vi "Disabled.vi"(7 "Robot Mode":T2, 10 "Match Info":T1={"Autonomous Elapsed Seconds"=0.0, "TeleOp Elapsed Seconds"=0.0, "Disabled Elapsed Seconds"=0.0, "Visited Autonomous"=FALSE, "Visited TeleOp"=FALSE, "Visited Disabled"=FALSE, "Autonomous Settings"={"Autonomous Style"=enum."Independent", "VI Refnum"=refnum}}, 11 "Call Context":T3) -> ()   [LabVIEW 2012]
doc: "This VI is called each time a disabled packet is received from the DS. It is often used to prepare for the next robot mode, to calibrate sensors, etc."
uses:
  <vilib>/Rock Robotics/WPI/DriverStation/WPI_DriverStationDerivedRobotMode.ctl
  <vilib>/Rock Robotics/WPI/DriverStation/WPI_DriverStationRobotMode2.ctl
  <vilib>/Rock Robotics/WPI/DriverStation/WPI_DriverStationMatch Info.ctl
  Robot Global Data.vi
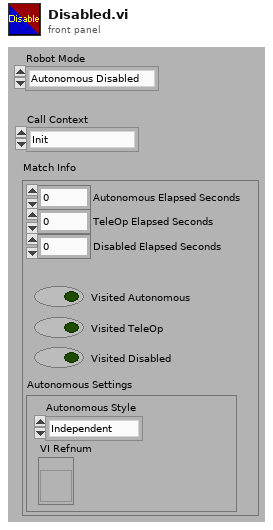
[diagram p1: front panel]
types:
  T1 = typedef "WPI_DriverStationMatch Info.ctl" = cluster{"Autonomous Elapsed Seconds":dbl, "TeleOp Elapsed Seconds":dbl, "Disabled Elapsed Seconds":dbl, "Visited Autonomous":bool, "Visited TeleOp":bool, "Visited Disabled":bool, "Autonomous Settings":cluster{"Autonomous Style":enum16{"Iterative", "Independent"}, "VI Refnum":refnum<vi>}}
  T2 = typedef "WPI_DriverStationRobotMode2.ctl" = enum16{"Autonomous Disabled", "Autonomous Enabled", "Teleop Disabled", "Teleop Enabled", "Timeout", "Finish", "Test Disabled", "Test Enabled"}
  T3 = typedef "WPI_DriverStationDerivedRobotMode.ctl" = enum16{"Init", "Execute", "Stop"}
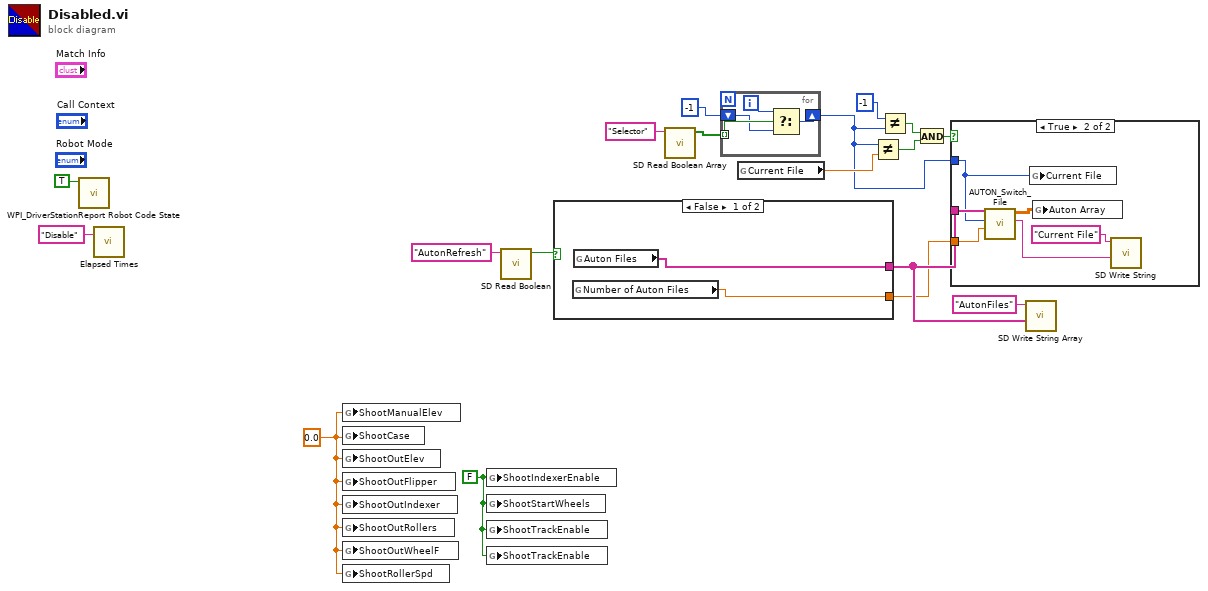
[diagram p0: block diagram]
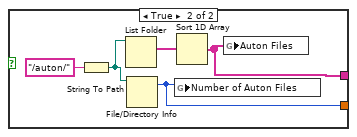
[diagram p3: hidden frame]
diagram:
  w13 = FALSE ("ShootIndexerEnable")
  w12 = 0.0 ("ShootCase")
  n1 = call <vilib>:"WPI_DriverStationReport Robot Code State.vi"("Disabled"=TRUE ("Autonomous")) -> ()  [unwired: 10 in, 1 out]
  n2 = call "Elapsed Times.vi"("Call Name"="Disable") -> ()  [unwired: 2 in, 1 out]
  n3 = global write "Robot Global Data.vi" "ShootManualElev"(w12) -> ()
  n4 = global write "Robot Global Data.vi" "ShootCase"(w12) -> ()
  n5 = global write "Robot Global Data.vi" "ShootOutElev"(w12) -> ()
  n6 = global write "Robot Global Data.vi" "ShootOutFlipper"(w12) -> ()
  n7 = global write "Robot Global Data.vi" "ShootOutIndexer"(w12) -> ()
  n8 = global write "Robot Global Data.vi" "ShootOutRollers"(w12) -> ()
  n9 = global write "Robot Global Data.vi" "ShootOutWheelF"(w12) -> ()
  n10 = global write "Robot Global Data.vi" "ShootRollerSpd"(w12) -> ()
  n11 = global write "Robot Global Data.vi" "ShootIndexerEnable"(w13) -> ()
  n12 = global write "Robot Global Data.vi" "ShootStartWheels"(w13) -> ()
  n13 = global write "Robot Global Data.vi" "ShootTrackEnable"(w13) -> ()
  n14 = global write "Robot Global Data.vi" "ShootTrackEnable"(w13) -> ()
  n15 = call <vilib>:"SD Read Boolean.vi"("Name"="AutonRefresh") -> ("Boolean"=w2:bool)  [unwired: 8 in, 2 out]
  n16 = case shown="False" w2 {
    tunnel: [w19 w22] -> w15
    tunnel: [w20 w21] -> w17
    frame False {
      n17 = global read "Robot Global Data.vi" "Number of Auton Files"() -> (w19:dbl)
      n18 = global read "Robot Global Data.vi" "Auton Files"() -> (w20:string[])
    }
    frame True {
      n19 = String To Path(string="/auton/") -> (path=w24:path)
      n20 = List Folder(path=w24) -> (filenames=w23:string[])  [unwired: 3 in, 3 out]
      n21 = File/Directory Info(path=w24) -> (size=w22:i64)  [unwired: 1 in, 6 out]
      n22 = global write "Robot Global Data.vi" "Number of Auton Files"(w22) -> ()
      n23 = Sort 1D Array(array=w23) -> (sorted array=w21:string[])
      n24 = global write "Robot Global Data.vi" "Auton Files"(w21) -> ()
    }
  }
  n25 = call <vilib>:"SD Read Boolean Array.vi"("Name"="Selector") -> ("Boolean Array"=w10:bool[])  [unwired: 8 in, 2 out]
  n26 = for {
    tunnel: w10 -> [w29] mode=indexing
    shift-right: [w27] -> w3
    shift-left: -1 -> [w26]
    i -> [w28]
    n27 = Select(t=w28, s=w29, f=w26) -> (s? t:f=w27:i32)
  }
  n28 = global read "Robot Global Data.vi" "Current File"() -> (w7:dbl)
  n29 = Not Equal?(x=w3, y=w7) -> (x != y?=w5:bool)
  n30 = Not Equal?(x=-1, y=w3) -> (x != y?=w6:bool)
  n31 = And(x=w6, y=w5) -> (x .and. y?=w4:bool)
  n32 = case shown="True" w4 {
    tunnel: w3 -> [_ w30]
    tunnel: w17 -> [_ w35]
    tunnel: w15 -> [_ w34]
    frame False {
    }
    frame True {
      n33 = call "AUTON_Switch_File.vi"("Number of Auton Files"=w34, "Auton File"=w30, "Auton Files"=w35) -> ("Current File"=w31:string, "Auton Array"=w33:dbl[][])  [unwired: 7 in]
      n34 = global write "Robot Global Data.vi" "Current File"(w30) -> ()
      n35 = global write "Robot Global Data.vi" "Auton Array"(w33) -> ()
      n36 = call <vilib>:"SD Write String.vi"("String"=w31, "Name"="Current File") -> ()  [unwired: 8 in, 2 out]
    }
  }
  n37 = call <vilib>:"SD Write String Array.vi"("String Array"=w17, "Name"="AutonFiles") -> ()  [unwired: 8 in, 2 out]
